vi "LoadInterface.vi"(0 "Application Interface in":refnum<class "Application Interface.lvclass">, 1 "application":refnum<class "Application.lvclass">, 2 "universalRobot":refnum<class "Universal Robot.lvclass">, 5 "error in (no error)":errorcluster) -> (14 "Application Interface out":refnum<class "Application Interface.lvclass">, 19 "error out":errorcluster)   [LabVIEW 2019, in "Application Interface.lvclass"]
uses:
  Application Interface.lvclass
  Application.lvclass
  Robot/Universal Robot/Universal Robot.lvclass
  Application Interface.lvclass/Application Interface.ctl
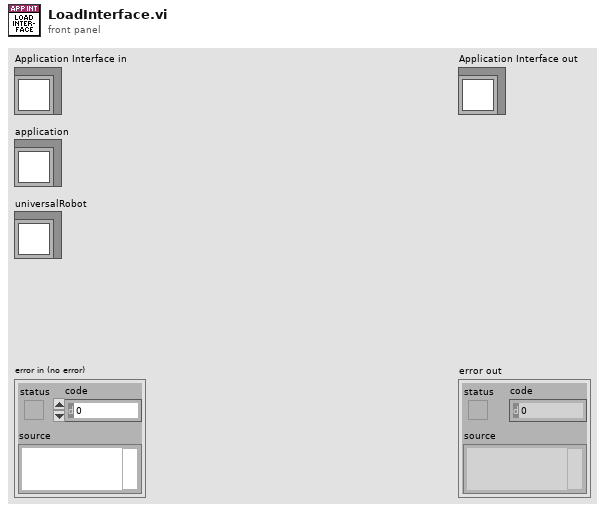
[diagram p1: front panel]
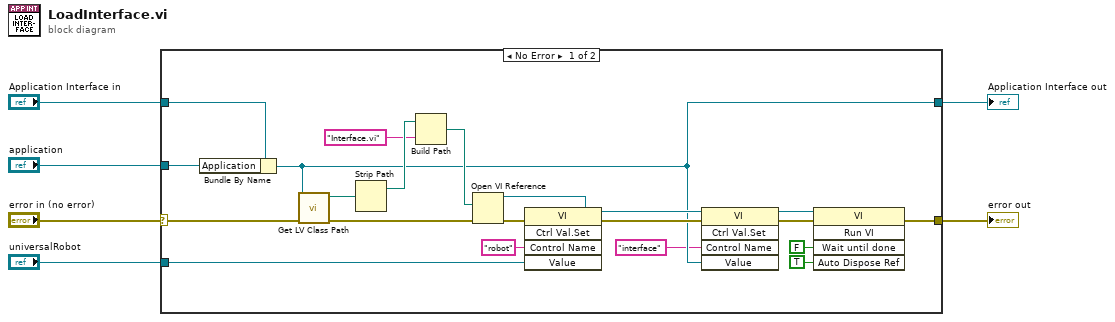
[diagram p0: block diagram]
diagram:
  n1 = case shown="No Error" "error in (no error)" {
    selector: "error in (no error)" -> [w27 w29]
    tunnel: [w7 w29] -> w5
    tunnel: [w14 w28] -> w3
    tunnel: "Application Interface in" -> [w17 w28]
    tunnel: "application" -> [w16 _]
    tunnel: "universalRobot" -> [w15 _]
    frame No Error {
      n2 = Bundle By Name(cluster=w17, "Application"=w16) -> (w14:refnum<class "Application Interface.lvclass">)
      n3 = call <vilib>:"Get LV Class Path.vi"("error in (no error)"=w27, "object"=w14) -> ("error out"=w23:errorcluster, "class path"=w26:path)  [unwired: 8 in]
      n4 = Strip Path(path=w26) -> (stripped path=w25:path)  [unwired: 1 out]
      n5 = Build Path(base path=w25, name or relative path="Interface.vi") -> (appended path=w22:path)
      n6 = Open VI Reference(vi path=w22, error in (no error)=w23) -> (vi reference=w21:refnum<vi>, error out=w20:errorcluster)  [unwired: 4 in]
      n7 = invoke class="VI" method="Ctrl Val.Set"(reference=w21, error in=w20, "Control Name"="robot", "Value"=w15) -> (reference out=w18:refnum<vi>, error out=w19:errorcluster)  [unwired: 1 in, 3 out]
      n8 = invoke class="VI" method="Ctrl Val.Set"(reference=w18, error in=w19, "Control Name"="interface", "Value"=w14) -> (reference out=w10:refnum<vi>, error out=w11:errorcluster)  [unwired: 1 in, 3 out]
      n9 = invoke class="VI" method="Run VI"(reference=w10, error in=w11, "Wait until done"=FALSE ("Wait Until Done"), "Auto Dispose Ref"=TRUE ("Auto Dispose Reference")) -> (error out=w7:errorcluster)  [unwired: 1 in, 4 out]
    }
    frame Error {
    }
  }
  "error out" <- w5
  "Application Interface out" <- w3
